vi "CMDstr.vi"(11 "Address":i8) -> (3 "CMD 2":string)   [LabVIEW 2015]
panel:
  out "CMD数组 2":u8[](array[numeric]) format="%.0x"
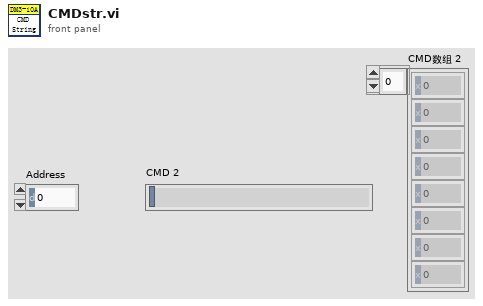
[diagram p1: front panel]
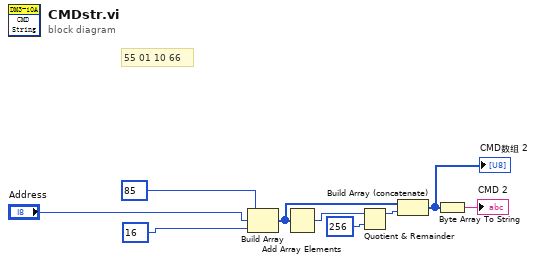
[diagram p0: block diagram]
diagram:
  # "55 01 10 66"
  n1 = Build Array(85, "Address", 16 ("元素")) -> (w4:i32[])
  n2 = Add Array Elements(numeric array=w4) -> (sum=w3:i32)
  n3 = Quotient & Remainder(x=w3, y=256) -> (x-y*floor(x/y)=w1:i32)  [unwired: 1 out]
  n4 = Build Array (concatenate)(w4, w1) -> (w9:i32[])
  "CMD数组 2" <- w9
  n5 = Byte Array To String(unsigned byte array=w9) -> (string=→"CMD 2":string)
